vi "Write.Initialize.vi"(8 "error in":errorcluster, 10 "PluginAPIs":T1, 11 "Settings":T2 {"Refs"."Data Reference" format="%.0x"}) -> (0 "error out":errorcluster, 3 "Write out":refnum<class "Write.lvclass">)   [LabVIEW 2023, in "Plugin Data Access Engine.lvlib" / "Write.lvclass"]
uses:
  Write.lvclass
  Write.lvclass/Write.ctl
  Program Files/NI/LVAddons/VS-CD-Plugin/1/Targets/win64/user.lib/PluginCore_v1.lvlibp/iPluginAPIs/iPluginAPIs.lvclass
  _PluginCore/Types/Plugin API.ctl
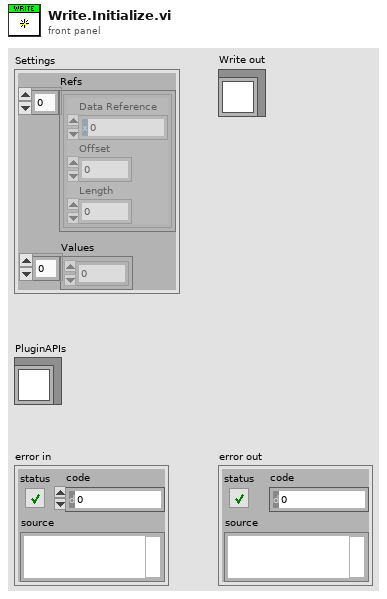
[diagram p1: front panel]
types:
  T1 = typedef "Plugin API.ctl" = refnum<class "iPluginAPIs.lvclass">
  T2 = cluster{"Refs":cluster{"Data Reference":i32, "Offset":u64, "Length":u64}[], "Values":dbl[]}
  T3 = cluster{"read mode":enum16{"polling", "blocking"}, "write mode":enum16{"polling", "blocking"}}
  T4 = cluster{"Data Reference":i32, "Offset":u64, "Length":u64}[]
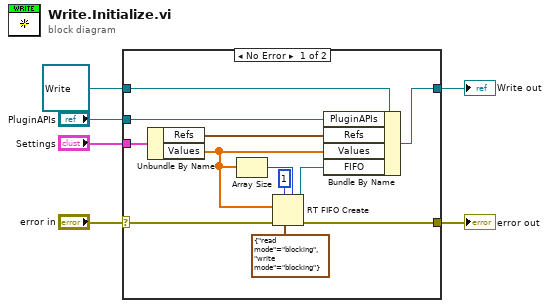
[diagram p0: block diagram]
diagram:
  n1 = case shown="No Error" "error in" {
    selector: "error in" -> [w11 w19]
    tunnel: [w18 w19] -> w6
    tunnel: refnum<class "Write.lvclass"> refnum ("Write in") -> [w13 w20]
    tunnel: [w12 w20] -> w4
    tunnel: "Settings" -> [w10 _]
    tunnel: "PluginAPIs" -> [w9 _]
    frame No Error {
      n2 = Unbundle By Name(w10) -> ("Refs"=w7:T4, "Values"=w8:dbl[])
      n3 = Array Size(array=w8) -> (size(s)=w15:i32)
      n4 = RT FIFO Create(1:w8, 3:w11, 4:u32 1 ("size (10)"), 6:w15, 7:T3 {"read mode"=enum."blocking", "write mode"=enum."blocking"} ("r/w modes (polling,polling)")) -> (8:w17:refnum<k33>, 11:w18:errorcluster)  [unwired: 3 in, 1 out]
      n5 = Bundle By Name(cluster=w13, "PluginAPIs"=w9, "Refs"=w7, "Values"=w8, "FIFO"=w17) -> (w12:refnum<class "Write.lvclass">)
    }
    frame Error {
    }
  }
  "error out" <- w6
  "Write out" <- w4
